vi "CAN_Send_command.vi"(4 "Numeric Request":u32, 5 "Read":refnum<k21>, 6 "CAN frame":T1 {"payload" format="%x"; "timestamp" format="%<%.7X\n%x>T"; "type" items=["CAN Data"=0, "CAN Remote"=1, "CAN Bus Error"=2, "CAN 2.0 Data"=8, "CAN FD Data"=16, "CAN FD+BRS Data"=24, "J1939 Data"=192, "Delay"=224, "Log Trigger"=225, "Start Trigger"=226]; "identifier" format="%x"}, 7 "Write":refnum<k21>) -> (0 "error out":errorcluster, 1 "Read":refnum<k21>, 2 "Write":refnum<k21>, 3 "cluster":T3 {"data[0]"."payload" format="%x"; "data[0]"."timestamp" format="%<%.7X\n%x>T"; "data[0]"."type" items=["CAN Data"=0, "CAN Remote"=1, "CAN Bus Error"=2, "CAN 2.0 Data"=8, "CAN FD Data"=16, "CAN FD+BRS Data"=24, "J1939 Data"=192, "Delay"=224, "Log Trigger"=225, "Start Trigger"=226]; "data[0]"."identifier" format="%x"; "data[1]"."payload" format="%x"; "data[1]"."timestamp" format="%<%.7X\n%x>T"; "data[1]"."type" items=["CAN Data"=0, "CAN Remote"=1, "CAN Bus Error"=2, "CAN 2.0 Data"=8, "CAN FD Data"=16, "CAN FD+BRS Data"=24, "J1939 Data"=192, "Delay"=224, "Log Trigger"=225, "Start Trigger"=226]; "data[1]"."identifier" format="%x"; "data[2]"."payload" format="%x"; "data[2]"."timestamp" format="%<%.7X\n%x>T"; "data[2]"."type" items=["CAN Data"=0, "CAN Remote"=1, "CAN Bus Error"=2, "CAN 2.0 Data"=8, "CAN FD Data"=16, "CAN FD+BRS Data"=24, "J1939 Data"=192, "Delay"=224, "Log Trigger"=225, "Start Trigger"=226]; "data[2]"."identifier" format="%x"; "data[3]"."payload" format="%x"; "data[3]"."timestamp" format="%<%.7X\n%x>T"; "data[3]"."type" items=["CAN Data"=0, "CAN Remote"=1, "CAN Bus Error"=2, "CAN 2.0 Data"=8, "CAN FD Data"=16, "CAN FD+BRS Data"=24, "J1939 Data"=192, "Delay"=224, "Log Trigger"=225, "Start Trigger"=226]; "data[3]"."identifier" format="%x"; "data[4]"."payload" format="%x"; "data[4]"."timestamp" format="%<%.7X\n%x>T"; "data[4]"."type" items=["CAN Data"=0, "CAN Remote"=1, "CAN Bus Error"=2, "CAN 2.0 Data"=8, "CAN FD Data"=16, "CAN FD+BRS Data"=24, "J1939 Data"=192, "Delay"=224, "Log Trigger"=225, "Start Trigger"=226]; "data[4]"."identifier" format="%x"; "data[5]"."payload" format="%x"; "data[5]"."timestamp" format="%<%.7X\n%x>T"; "data[5]"."type" items=["CAN Data"=0, "CAN Remote"=1, "CAN Bus Error"=2, "CAN 2.0 Data"=8, "CAN FD Data"=16, "CAN FD+BRS Data"=24, "J1939 Data"=192, "Delay"=224, "Log Trigger"=225, "Start Trigger"=226]; "data[5]"."identifier" format="%x"; "data[6]"."payload" format="%x"; "data[6]"."timestamp" format="%<%.7X\n%x>T"; "data[6]"."type" items=["CAN Data"=0, "CAN Remote"=1, "CAN Bus Error"=2, "CAN 2.0 Data"=8, "CAN FD Data"=16, "CAN FD+BRS Data"=24, "J1939 Data"=192, "Delay"=224, "Log Trigger"=225, "Start Trigger"=226]; "data[6]"."identifier" format="%x"; "data[7]"."payload" format="%x"; "data[7]"."timestamp" format="%<%.7X\n%x>T"; "data[7]"."type" items=["CAN Data"=0, "CAN Remote"=1, "CAN Bus Error"=2, "CAN 2.0 Data"=8, "CAN FD Data"=16, "CAN FD+BRS Data"=24, "J1939 Data"=192, "Delay"=224, "Log Trigger"=225, "Start Trigger"=226]; "data[7]"."identifier" format="%x"; "data[8]"."payload" format="%x"; "data[8]"."timestamp" format="%<%.7X\n%x>T"; "data[8]"."type" items=["CAN Data"=0, "CAN Remote"=1, "CAN Bus Error"=2, "CAN 2.0 Data"=8, "CAN FD Data"=16, "CAN FD+BRS Data"=24, "J1939 Data"=192, "Delay"=224, "Log Trigger"=225, "Start Trigger"=226]; "data[8]"."identifier" format="%x"})   [LabVIEW 2023]
uses:
  <vilib>/xnet/xnet.llb/XNET Frame CAN.ctl
  <vilib>/xnet/xnet.llb/XNET Frame Type CAN.ctl
  <vilib>/xnet/xnet.llb/XNET Write (Frame CAN).vi
  <vilib>/xnet/xnet.llb/XNET Read (Frame CAN).vi
panel:
  in  "error in (no error)":errorcluster
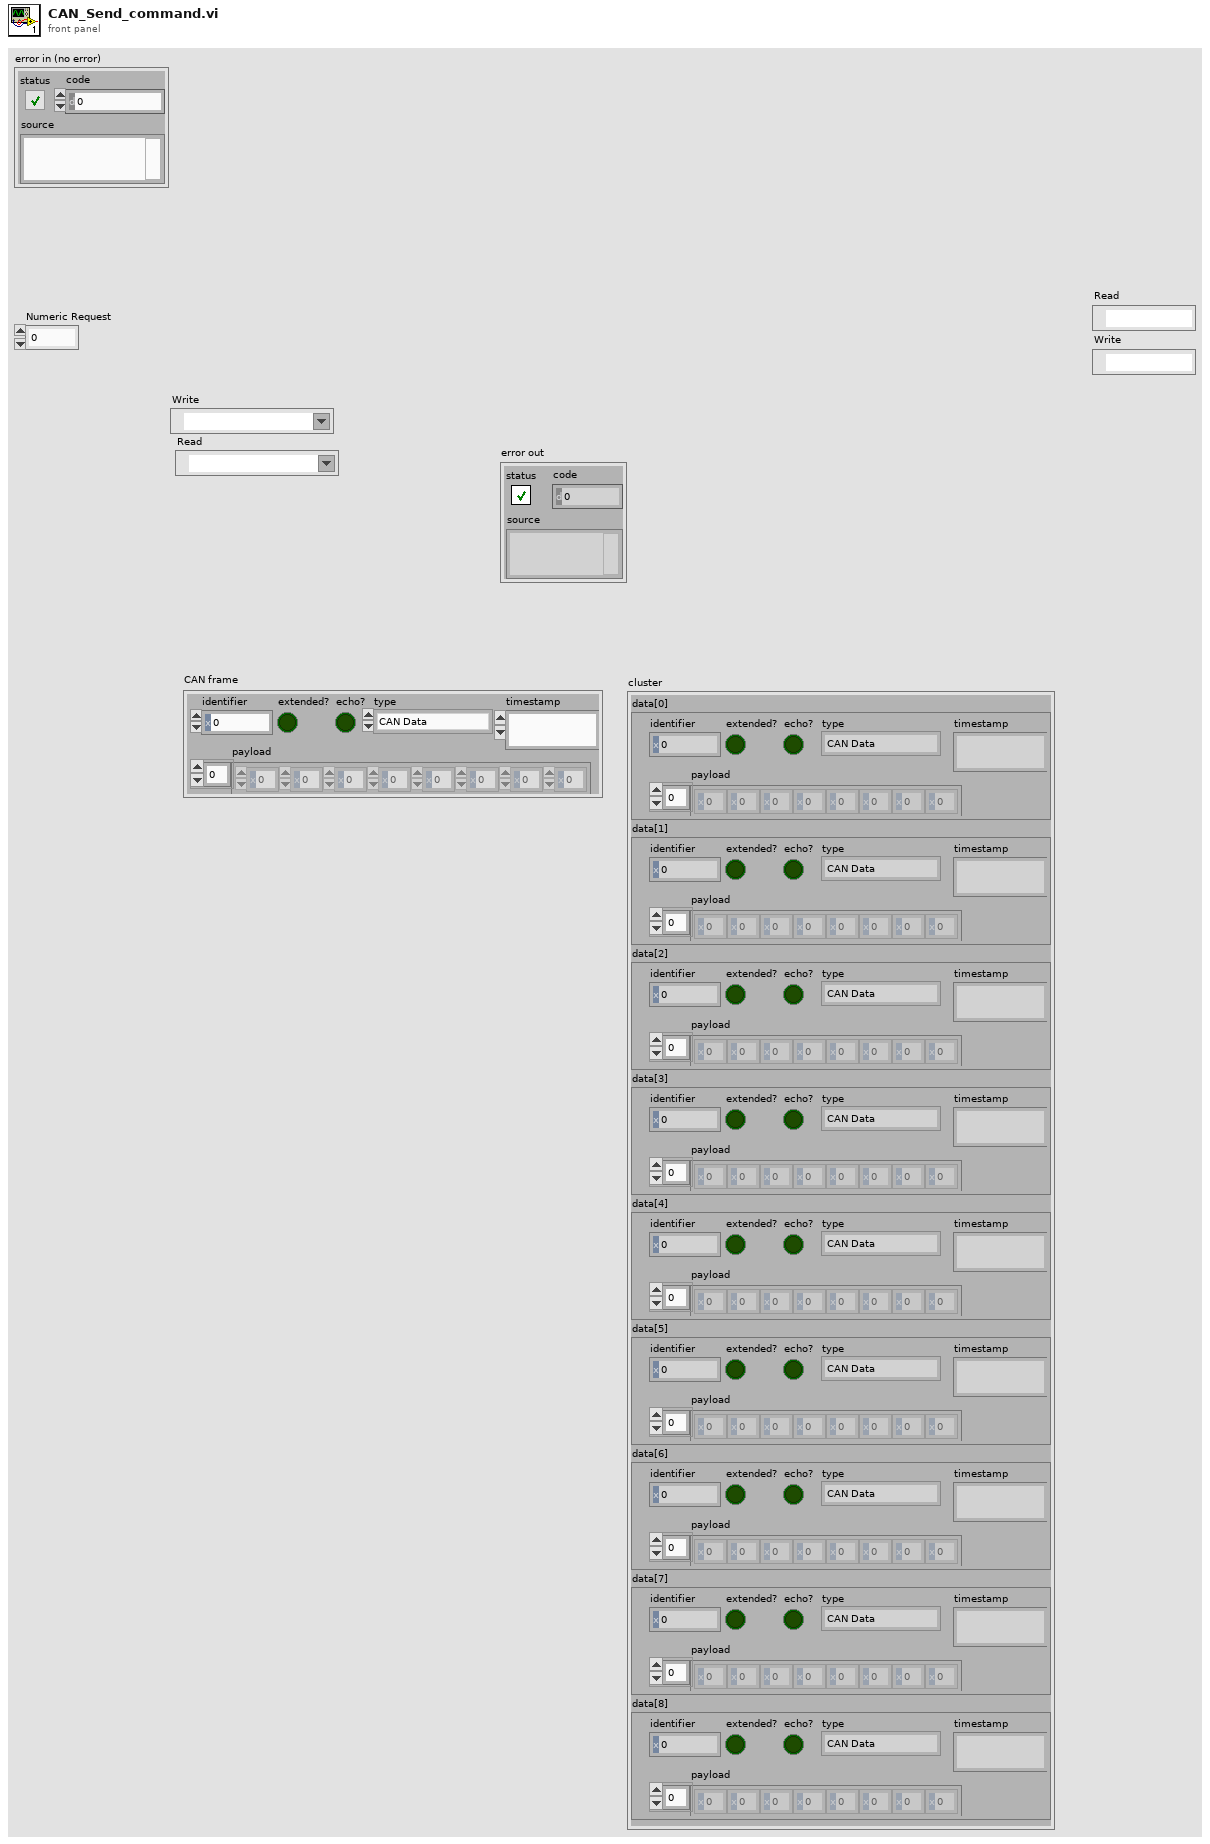
[diagram p1: front panel]
types:
  T1 = typedef "XNET Frame CAN.ctl" = cluster{"timestamp":timestamp, "payload":u8[], "identifier":u32, "type":T2, "extended?":bool, "echo?":bool}
  T2 = typedef "XNET Frame Type CAN.ctl" = u8
  T3 = cluster{"data[0]":T1, "data[1]":T1, "data[2]":T1, "data[3]":T1, "data[4]":T1, "data[5]":T1, "data[6]":T1, "data[7]":T1, "data[8]":T1}
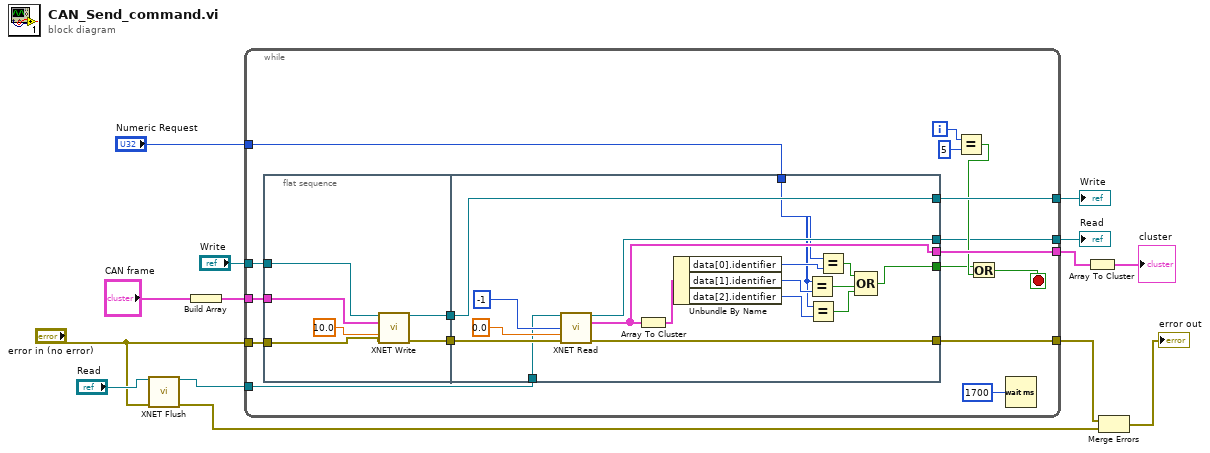
[diagram p0: block diagram]
diagram:
  n1 = call <vilib>:"XNET Flush.vi"("session in"="Read", "error in (no error)"="error in (no error)") -> ("session out"=w6:refnum<k21>, "error out"=w2:errorcluster)  [unwired: 12 in]
  n2 = Build Array("CAN frame") -> (w11:T1[])
  n3 = while {
    tunnel: w6 -> [w19]
    tunnel: "Write" -> [w31]
    tunnel: [w28] -> w3
    tunnel: [w27] -> w14
    tunnel: w11 -> [w26]
    tunnel: [w25] -> w9
    tunnel: [w20] -> w8
    tunnel: "Numeric Request" -> [w17]
    tunnel: "error in (no error)" -> [w16]
    i -> [w23]
    stop <- w18 stop-if-true
    n4 = flat-sequence {
      tunnel: w31 -> [w37]
      tunnel: [w35] -> w30
      tunnel: w26 -> [w34]
      tunnel: [w33] -> w24
      tunnel: w16 -> [w32]
      tunnel: w30 -> [w52]
      tunnel: w19 -> [w51]
      tunnel: [w50] -> w28
      tunnel: [w49] -> w27
      tunnel: [w48] -> w20
      tunnel: [w47] -> w25
      tunnel: w24 -> [w47]
      tunnel: w17 -> [w38]
      tunnel: [w42] -> w15
      frame #0 {
        n5 = call-poly <vilib>:"XNET Write.vi"("session in"=w37, "data"=w34, "timeout (10)"=10.0, "error in (no error)"=w32) -> ("session out"=w33:refnum<k21>, "error out"=w35:errorcluster)  [unwired: 10 in]
      }
      frame #1 {
        n6 = call-poly <vilib>:"XNET Read.vi"("session in"=w51, "number to read (-1)"=-1, "timeout (0)"=0.0, "error in (no error)"=w52) -> ("session out"=w48:refnum<k21>, "data"=w49:T1[], "error out"=w50:errorcluster)  [unwired: 8 in, 1 out]
        n7 = Array To Cluster(array=w49) -> (cluster=w46:T3)
        n8 = Unbundle By Name(w46) -> ("data[0].identifier"=w39:u32, "data[1].identifier"=w41:u32, "data[2].identifier"=w40:u32)
        n9 = Equal?(x=w38, y=w41) -> (x = y?=w45:bool)
        n10 = Equal?(x=w38, y=w40) -> (x = y?=w44:bool)
        n11 = Equal?(x=w38, y=w39) -> (x = y?=w43:bool)
        n12 = Compound Arithmetic op=OR(w43, w45, w44) -> (w42:bool)
      }
    }
    n13 = Equal?(x=w23, y=5) -> (x = y?=w22:bool)
    n14 = Or(x=w15, y=w22) -> (x .or. y?=w18:bool)
    n15 = Wait (ms)(milliseconds to wait=u32 1700) -> ()  [unwired: 1 out]
  }
  "Read" <- w8
  "Write" <- w9
  n16 = Array To Cluster(array=w14) -> (cluster=→"cluster":T3)
  n17 = Merge Errors(w3, w2) -> (→"error out":errorcluster)
